vi "Arm Hardware.vi"(8 "error in (no error)":errorcluster, 11 "DAQmx Digitizer in":refnum<class "DAQmx Digitizer.lvclass">) -> (0 "error out":errorcluster, 3 "DAQmx Digitizer out":refnum<class "DAQmx Digitizer.lvclass">)   [LabVIEW 2021, in "DAQmx Digitizer.lvclass"]
uses:
  DAQmx Digitizer.lvclass
  DAQmx Digitizer.lvclass/DAQmx Digitizer.ctl
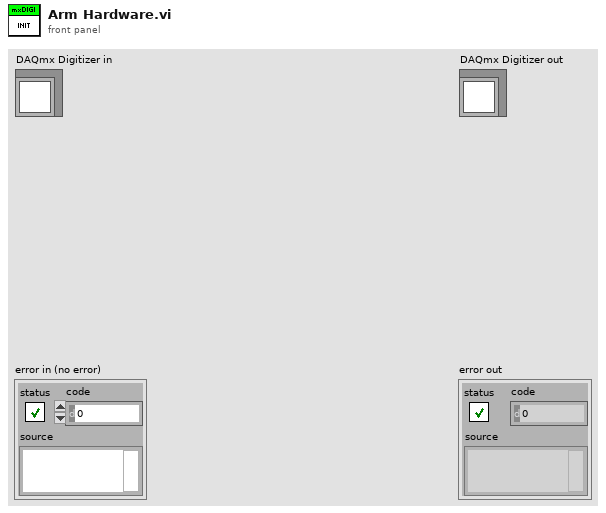
[diagram p1: front panel]
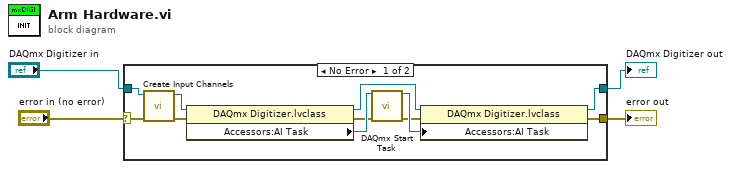
[diagram p0: block diagram]
diagram:
  n1 = case shown="No Error" "error in (no error)" {
    selector: "error in (no error)" -> [w5 w17]
    tunnel: [w6 w17] -> w3
    tunnel: [w7 w16] -> w1
    tunnel: "DAQmx Digitizer in" -> [w15 w16]
    frame No Error {
      n2 = call-dynamic "Create Input Channels.vi"("error in (no error)"=w5, "DAQmx Digitizer in"=w15) -> ("error out"=w13:errorcluster, "DAQmx Digitizer out"=w14:refnum<class "DAQmx Digitizer.lvclass">)  [unwired: 8 in]
      n3 = property class="DAQmx Digitizer.lvclass"(reference=w14, error in=w13) -> (reference out=w8:refnum<class "DAQmx Digitizer.lvclass">, error out=w11:errorcluster, "Accessors:AI Task"=w12:refnum<k21>)
      n4 = call <vilib>:"DAQmx Start Task.vi"("task/channels in"=w12, "error in"=w11) -> ("task out"=w10:refnum<k21>, "error out"=w9:errorcluster)  [unwired: 12 out]
      n5 = property class="DAQmx Digitizer.lvclass"(reference=w8, error in=w9, "Accessors:AI Task"=w10) -> (reference out=w7:refnum<class "DAQmx Digitizer.lvclass">, error out=w6:errorcluster)
    }
    frame Error {
    }
  }
  "error out" <- w3
  "DAQmx Digitizer out" <- w1
